vi "TCPIP_PS_CONTROL.vi"() -> ()   [LabVIEW 2016]
uses:
  typedefs/states.ctl
panel:
  out "Rcv'd Data":string
  in  "stop":bool
  in  "Slew Rate [T/Min]":dbl=1.0 caption="(7.055) Max)" min=0.001 max=50.0 step=0.01 format="%.3f"
  in  "Setpoint [T]":dbl caption="(34.68) Max)" min=-34.679602421022246 max=34.679602421022246 format="%.5f"
  in  "Pause":bool
  out "Field [T]":dbl caption="Current [kA]" format="%.5f"
  in  "Units":enum32{"tesla", "kAmps"}(radio) caption="tesla            kAmps"
  in  "Ramp":bool
  in  "TCP/IP Port":u16=6341
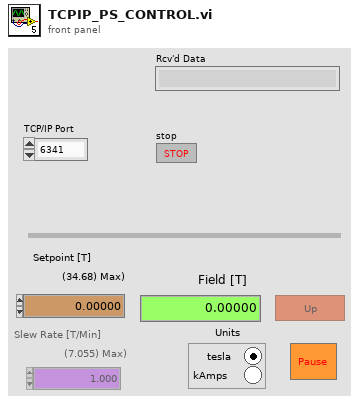
[diagram p1: front panel]
types:
  T1 = typedef "states.ctl" = enum16{"Initialize", "Status Check", "Read Data", "Write Data", "Stop"}
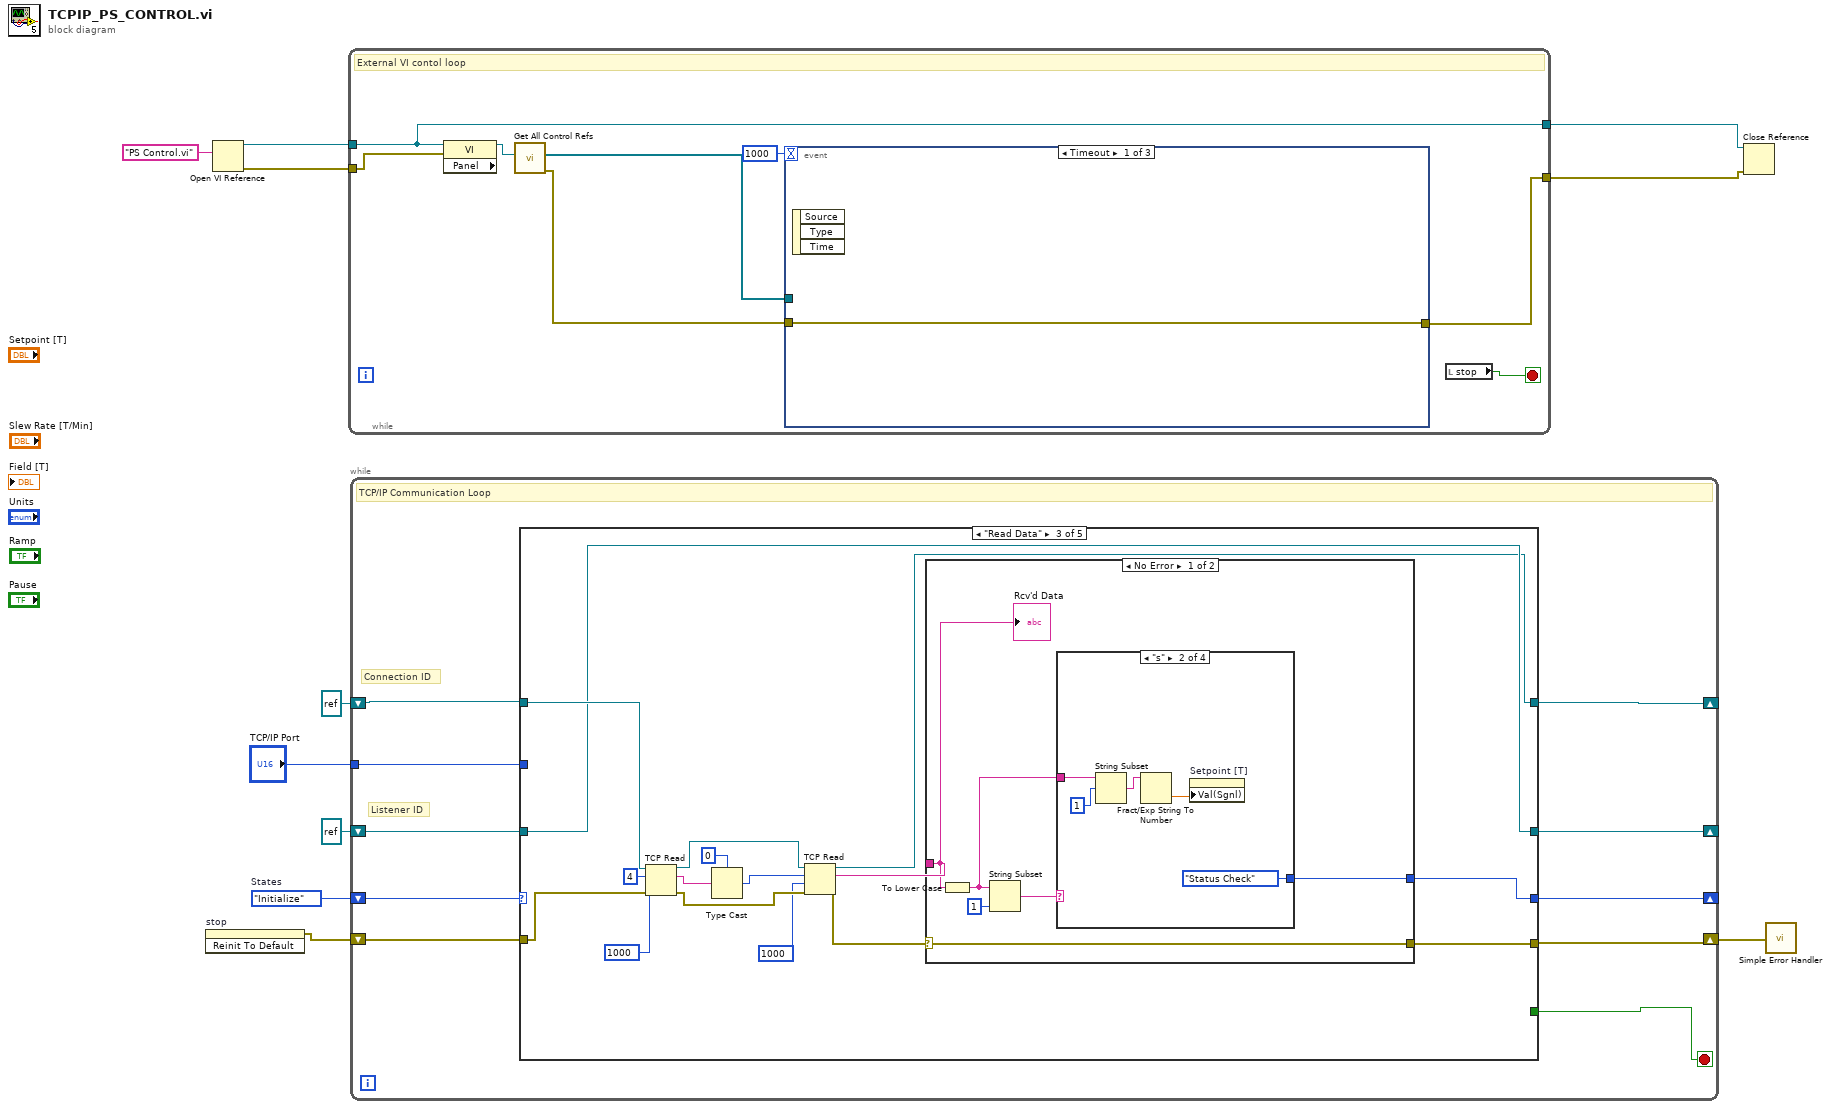
[diagram p0: block diagram]
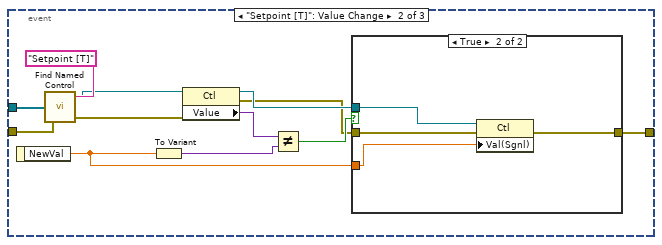
[diagram p2: hidden frame]
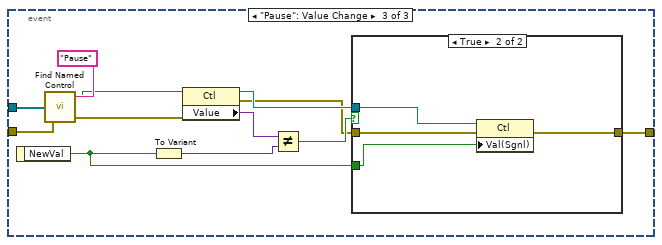
[diagram p4: hidden frame]
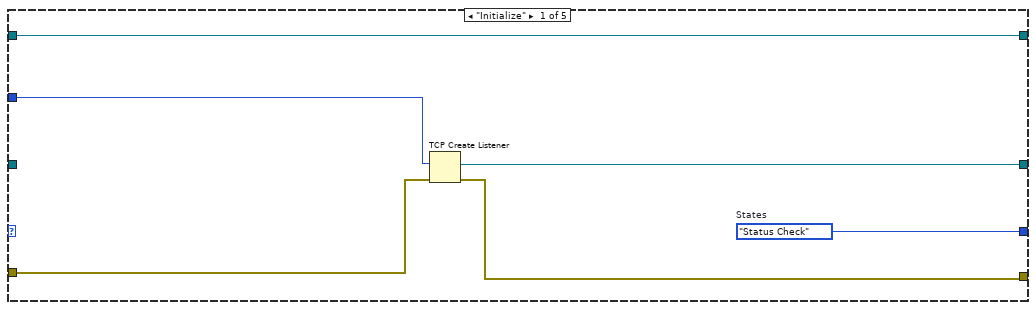
[diagram p6: hidden frame]
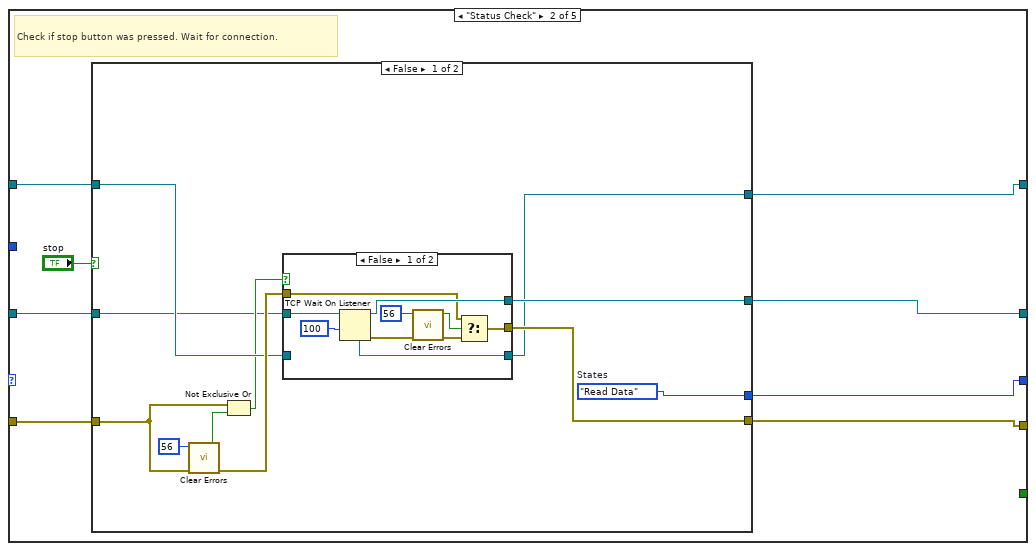
[diagram p7: hidden frame]
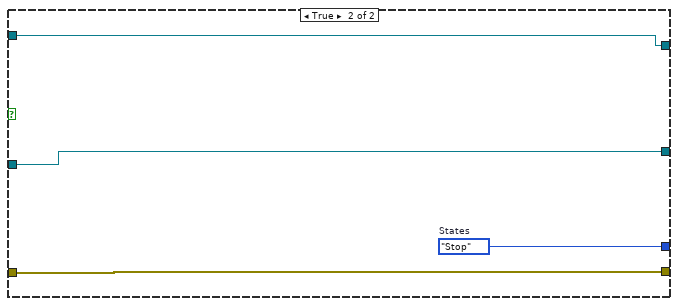
[diagram p9: hidden frame]
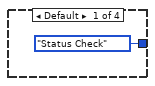
[diagram p10: hidden frame]
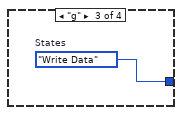
[diagram p11: hidden frame]
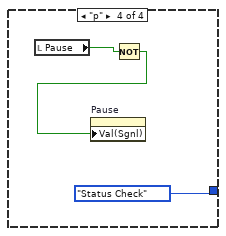
[diagram p12: hidden frame]
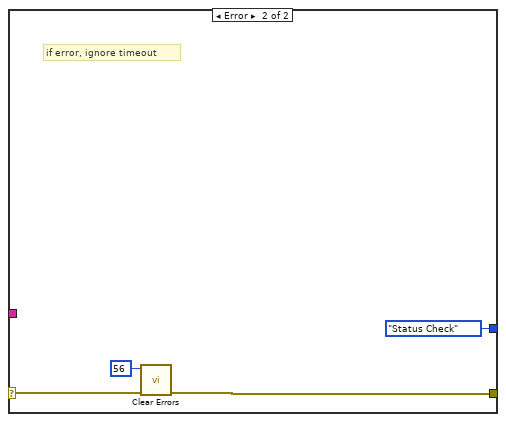
[diagram p13: hidden frame]
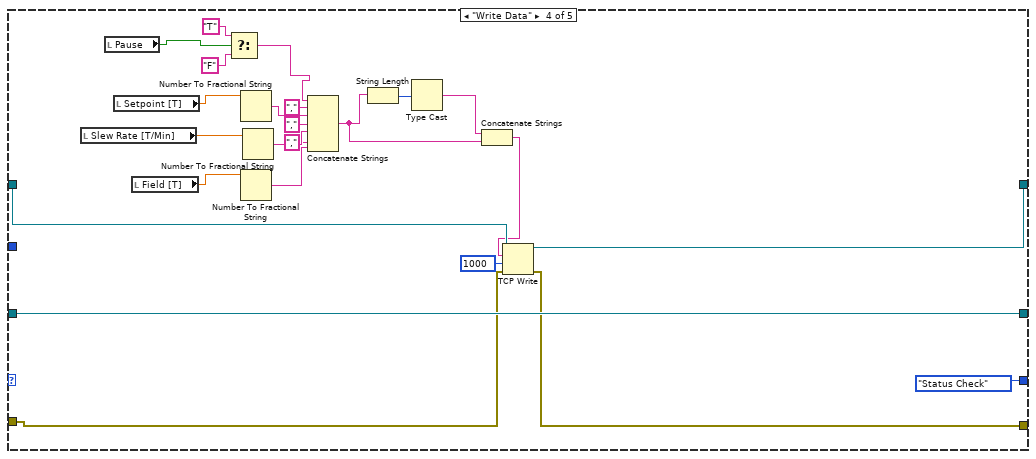
[diagram p14: hidden frame]
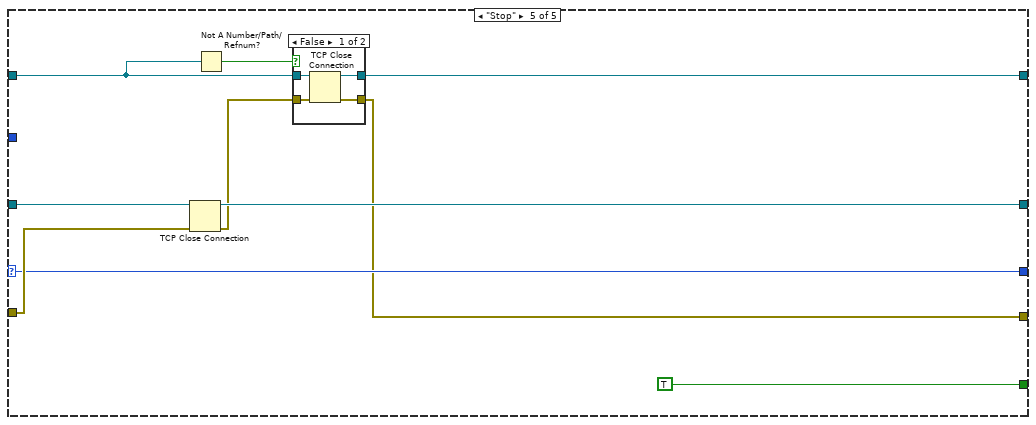
[diagram p15: hidden frame]
diagram:
  w9 = states."Initialize"  # States
  n1 = invoke on="stop" class="Bool (strict)" method="Reinit To Default"() -> (error out=w8:errorcluster)  [unwired: 3 in, 2 out]
  n2 = Open VI Reference(vi path="PS Control.vi") -> (vi reference=w7:refnum<vi>, error out=w6:errorcluster)  [unwired: 5 in]
  n3 = while {
    tunnel: w7 -> [w16]
    tunnel: w6 -> [w19]
    tunnel: [w16] -> w5
    tunnel: [w15] -> w4
    stop <- w14 stop-if-true
    # "External VI contol loop"
    n4 = property class="VI" props=["Panel"](reference=w16, error in=w19) -> (reference out=w18:refnum<vi>)  [unwired: 2 out]
    n5 = call "Get All Control Refs.vi"("vi reference"=w18) -> ("All Controls"=w12:refnum<vi>[], "error out"=w17:errorcluster)  [unwired: 5 in, 1 out]
    n6 = event shown="[0] Timeout" {
      selector: _ -> [_ _ _]
      dyn-events: _ -> [_ _ _]
      timeout: 1000 -> [_ _ _]
      tunnel: w17 -> [w20 w32 w49]
      tunnel: [w20 w23 w40] -> w15
      tunnel: w12 -> [_ w22 w39]
      event Timeout {
        n7 = event-data() -> ()  [unwired: 1 in, 3 out]
      }
      event "Setpoint [T]": Value Change {
        n8 = event-data() -> ("NewVal"=w25:dbl)  [unwired: 1 in]
        n9 = call "Find Named Control.vi"("error in"=w32, "All Controls"=w22, "Control Name"="Setpoint [T]") -> ("error out"=w30:errorcluster, "Ctl Refnum"=w21:refnum<vi>)  [unwired: 1 out]
        n10 = To Variant(anything=w25) -> (Variant=w28:variant)
        n11 = property class="Ctl"(reference=w21, error in=w30) -> (reference out=w26:refnum<vi>, error out=w24:errorcluster, "Value"=w29:variant)
        n12 = Not Equal?(x=w29, y=w28) -> (x != y?=w27:bool)
        n13 = case shown="True" w27 {
          tunnel: w26 -> [_ w37]
          tunnel: w25 -> [_ w36]
          tunnel: w24 -> [w33 w35]
          tunnel: [w33 w34] -> w23
          frame False {
          }
          frame True {
            n14 = property class="Ctl"(reference=w37, error in=w35, "Val(Sgnl)"=w36) -> (error out=w34:errorcluster)  [unwired: 1 out]
          }
        }
      }
      event "Pause": Value Change {
        n15 = event-data() -> ("NewVal"=w42:bool)  [unwired: 1 in]
        n16 = call "Find Named Control.vi"("error in"=w49, "All Controls"=w39, "Control Name"="Pause") -> ("error out"=w47:errorcluster, "Ctl Refnum"=w38:refnum<vi>)  [unwired: 1 out]
        n17 = To Variant(anything=w42) -> (Variant=w45:variant)
        n18 = property class="Ctl"(reference=w38, error in=w47) -> (reference out=w43:refnum<vi>, error out=w41:errorcluster, "Value"=w46:variant)
        n19 = Not Equal?(x=w46, y=w45) -> (x != y?=w44:bool)
        n20 = case shown="True" w44 {
          tunnel: w43 -> [_ w54]
          tunnel: w42 -> [_ w53]
          tunnel: w41 -> [w50 w52]
          tunnel: [w50 w51] -> w40
          frame False {
          }
          frame True {
            n21 = property class="Ctl"(reference=w54, error in=w52, "Val(Sgnl)"=w53) -> (error out=w51:errorcluster)  [unwired: 1 out]
          }
        }
      }
    }
    n22 = local read "stop"() -> (w14:bool)
  }
  n23 = while {
    tunnel: "TCP/IP Port" -> [w63]
    shift-right: [w56] -> _
    shift-left: w9 -> [w64]
    shift-right: [w61] -> w10
    shift-left: w8 -> [w62]
    shift-right: [w60] -> _
    shift-left: refnum<k5> refnum ("listener ID") -> [w59]
    shift-right: [w58] -> _
    shift-left: refnum<k5> refnum ("listener ID") -> [w57]
    stop <- w55 stop-if-true
    # "Connection ID"
    # "Listener ID"
    # "TCP/IP Communication Loop"
    n24 = case shown="\"Read Data\"" w64 {
      selector: w64 -> [_ _ _ _ w173]
      tunnel: w63 -> [w68 _ _ _ _]
      tunnel: w62 -> [w70 w78 w122 w162 w175]
      tunnel: [w69 w75 w114 w161 w167] -> w61
      tunnel: [w67 w74 w112 w166 w172] -> w60
      tunnel: [_ _ _ _ TRUE ("stop")] -> w55
      tunnel: w59 -> [_ w76 w112 w166 w174]
      tunnel: [w66 w71 w111 w163 w170] -> w58
      tunnel: w57 -> [w66 w72 w113 w164 w169]
      tunnel: [w65 w73 w107 states."Status Check" ("States") w173] -> w56
      frame "Initialize" {
        w65 = states."Status Check"  # States
        n25 = TCP Create Listener(8:w70, 10:w68) -> (0:w69:errorcluster, 3:w67:refnum<k5>)  [unwired: 3 in, 1 out]
      }
      frame "Status Check" {
        # "Check if stop button was pressed. Wait for connection."
        n26 = case shown="False" "stop" {
          tunnel: [w87 w106] -> w73
          tunnel: [w81 w104] -> w74
          tunnel: w78 -> [w83 w105]
          tunnel: [w86 w105] -> w75
          tunnel: w76 -> [w82 w104]
          tunnel: w72 -> [w88 w103]
          tunnel: [w80 w103] -> w71
          frame False {
            w87 = states."Read Data"  # States
            n27 = call <vilib>:"Clear Errors.vi"("error in (no error)"=w83, "specific error code to clear (0: all)"=56) -> ("error out"=w89:errorcluster, "specific error cleared?"=w84:bool)  [unwired: 4 in]
            n28 = Not Exclusive Or(1:w84, 2:w83) -> (0:w85:bool)
            n29 = case shown="False" w85 {
              tunnel: w89 -> [w92 w102]
              tunnel: [w91 w102] -> w86
              tunnel: w88 -> [_ w101]
              tunnel: [w98 w100] -> w81
              tunnel: w82 -> [w97 w100]
              tunnel: [w96 w101] -> w80
              frame False {
                n30 = TCP Wait On Listener(9:100 ("timeout ms (wait forever: -1)"), 11:w97) -> (0:w95:errorcluster, 3:w98:refnum<k5>, 4:w96:refnum<k5>)  [unwired: 2 in, 2 out]
                n31 = call <vilib>:"Clear Errors.vi"("error in (no error)"=w95, "specific error code to clear (0: all)"=56) -> ("error out"=w93:errorcluster, "specific error cleared?"=w94:bool)  [unwired: 4 in]
                n32 = Select(t=w92, s=w94, f=w93) -> (s? t:f=w91:errorcluster)
              }
              frame True {
              }
            }
          }
          frame True {
            w106 = states."Stop"  # States
          }
        }
      }
      frame "Read Data" {
        n33 = TCP Read(connection ID=w113, bytes to read=4, error in (no error)=w122, 9:1000 ("timeout ms (25000)")) -> (connection ID out=w117:refnum<k5>, data out=w120:string, error out=w116:errorcluster)  [unwired: 1 in]
        n34 = Type Cast(type=u8 0, x=w120) -> (*(type *) &x=w118:u8)
        n35 = TCP Read(connection ID=w117, bytes to read=w118, error in (no error)=w116, 9:1000 ("timeout ms (25000)")) -> (connection ID out=w111:refnum<k5>, data out=w110:string, error out=w115:errorcluster)  [unwired: 1 in]
        n36 = case shown="No Error" w115 {
          selector: w115 -> [w126 w141]
          tunnel: [w126 w139] -> w114
          tunnel: w110 -> [w128 _]
          tunnel: [w123 states."Status Check" ("States")] -> w107
          frame No Error {
            n37 = To Lower Case(string=w128) -> (all lower case string=w125:string)
            n38 = String Subset(string=w125, length (rest)=1 ("length (rest)")) -> (substring=w124:string)  [unwired: 1 in]
            n39 = case shown="\"s\"" w124 {
              tunnel: w125 -> [_ w134 _ _]
              tunnel: [states."Status Check" ("States") states."Status Check" ("States") w135 states."Status Check" ("States")] -> w123
              frame Default {
              }
              frame "s" {
                n40 = String Subset(string=w134, offset (0)=1) -> (substring=w132:string)  [unwired: 1 in]
                n41 = Fract/Exp String To Number(string=w132) -> (number=w131:dbl)  [unwired: 3 in, 1 out]
                n42 = property on="Setpoint [T]" class="DigNum (strict)"("Val(Sgnl)"=w131) -> ()  [unwired: 2 in, 2 out]
              }
              frame "g" {
                w135 = states."Write Data"  # States
              }
              frame "p" {
                n43 = local read "Pause"() -> (w138:bool)
                n44 = Not(x=w138) -> (.not. x?=w137:bool)
                n45 = property on="Pause" class="Bool (strict)"("Val(Sgnl)"=w137) -> ()  [unwired: 2 in, 2 out]
              }
            }
            "Rcv'd Data" <- w128
          }
          frame Error {
            # "if error, ignore timeout"
            n46 = call <vilib>:"Clear Errors.vi"("error in (no error)"=w141, "specific error code to clear (0: all)"=56) -> ("error out"=w139:errorcluster)  [unwired: 4 in, 1 out]
          }
        }
      }
      frame "Write Data" {
        n47 = local read "Slew Rate [T/Min]"() -> (w159:dbl)
        n48 = local read "Pause"() -> (w153:bool)
        n49 = local read "Setpoint [T]"() -> (w160:dbl)
        n50 = local read "Field [T]"() -> (w144:dbl)
        n51 = Select(t="T", s=w153, f="F") -> (s? t:f=w149:string)
        n52 = Number To Fractional String(number=w160) -> (F-format string=w158:string)  [unwired: 3 in]
        n53 = Number To Fractional String(number=w144) -> (F-format string=w143:string)  [unwired: 3 in]
        n54 = Number To Fractional String(number=w159) -> (F-format string=w147:string)  [unwired: 3 in]
        n55 = Concatenate Strings(w149, "," ("string"), w158, "," ("string"), w147, "," ("string"), w143) -> (w155:string)
        n56 = String Length(string=w155) -> (length=w157:i32)
        n57 = Type Cast(x=w157) -> (*(type *) &x=w156:string)  [unwired: 1 in]
        n58 = Concatenate Strings(w156, w155) -> (w154:string)
        n59 = TCP Write(connection ID=w164, data in=w154, error in (no error)=w162, 9:1000 ("timeout ms (25000)")) -> (connection ID out=w163:refnum<k5>, error out=w161:errorcluster)  [unwired: 1 out]
      }
      frame "Stop" {
        n60 = TCP Close Connection(connection ID=w174, error in (no error)=w175) -> (connection ID out=w172:refnum<k5>, error out=w168:errorcluster)  [unwired: 1 in]
        n61 = Not A Number/Path/Refnum?(number/path/refnum=w169) -> (NaN/Path/Refnum?=w171:bool)
        n62 = case shown="False" w171 {
          tunnel: [w180 w181] -> w170
          tunnel: w169 -> [w179 w181]
          tunnel: w168 -> [w178 w182]
          tunnel: [w177 w182] -> w167
          frame False {
            n63 = TCP Close Connection(connection ID=w179, error in (no error)=w178) -> (connection ID out=w180:refnum<k5>, error out=w177:errorcluster)  [unwired: 1 in]
          }
          frame True {
          }
        }
      }
    }
  }
  n64 = Close Reference(reference=w5, error in (no error)=w4) -> ()  [unwired: 1 out]
  n65 = call <vilib>:"Simple Error Handler.vi"("error in (no error)"=w10) -> ()  [unwired: 4 in, 5 out]
